vi "Color sensor - main.vi"() -> ()   [LabVIEW 2022 SP3]
uses:
  Power mode.ctl
panel:
  in  "RED MIN 2%":dbl=193.0
  in  "RED MAX 2%":dbl=1715.0
  in  "BLUE MIN 2%":dbl=221.0
  in  "GREEN MIN 2%":dbl=158.0
  in  "GREEN MAX 2%":dbl=1834.0
  in  "BLUE MAX 2%":dbl=2778.0
  in  "RED MIN 20%":dbl=1939.0
  in  "RED MAX 20%":dbl=17200.0
  in  "BLUE MIN 20%":dbl=2215.0
  in  "GREEN MIN 20%":dbl=1585.0
  in  "GREEN MAX 20%":dbl=18400.0
  in  "BLUE MAX 20%":dbl=27800.0
  in  "Power mode":T1=enum."100%"
  in  "GREEN Sensitivity":dbl(slide)=1.0 scale=0.0..2.0
  in  "BLUE Sensitivity":dbl(slide)=1.0 scale=0.0..2.0
  in  "RED Sensitivity":dbl(slide)=1.0 scale=0.0..2.0
  in  "RGB TARGET":u32(colorbox)=16448250
  out "TARGET B":dbl=250.0 caption="B" format="%#_3g"
  out "TARGET G":dbl=250.0 caption="G" format="%#_3g"
  out "TARGET R":dbl=250.0 caption="R" format="%#_3g"
  out "G":dbl format="%#_3g"
  out "R":dbl format="%#_3g"
  out "B":dbl format="%#_3g"
  in  "GREEN MAX 100%":dbl=92000.0
  in  "GREEN MIN 100%":dbl=7910.0
  in  "BLUE MAX 100%":dbl=139000.0
  in  "BLUE MIN 100%":dbl=11060.0
  in  "RED MAX 100%":dbl=85900.0
  in  "RED MIN 100%":dbl=9680.0
  out "RGB OUTPUT":u32(colorbox)=262914
  out "GREEN Frequency":dbl
  out "CLEAR Frequency":dbl
  out "BLUE Frequency":dbl
  in  "stop":bool
  out "RED Frequency":dbl
  out "Color Chart":T2(graph)={"Scalar"=10835.410120273053, "Scalar"=12236.906510034263, "Scalar"=31123.560535325243, "Scalar"=8833.141948591114}
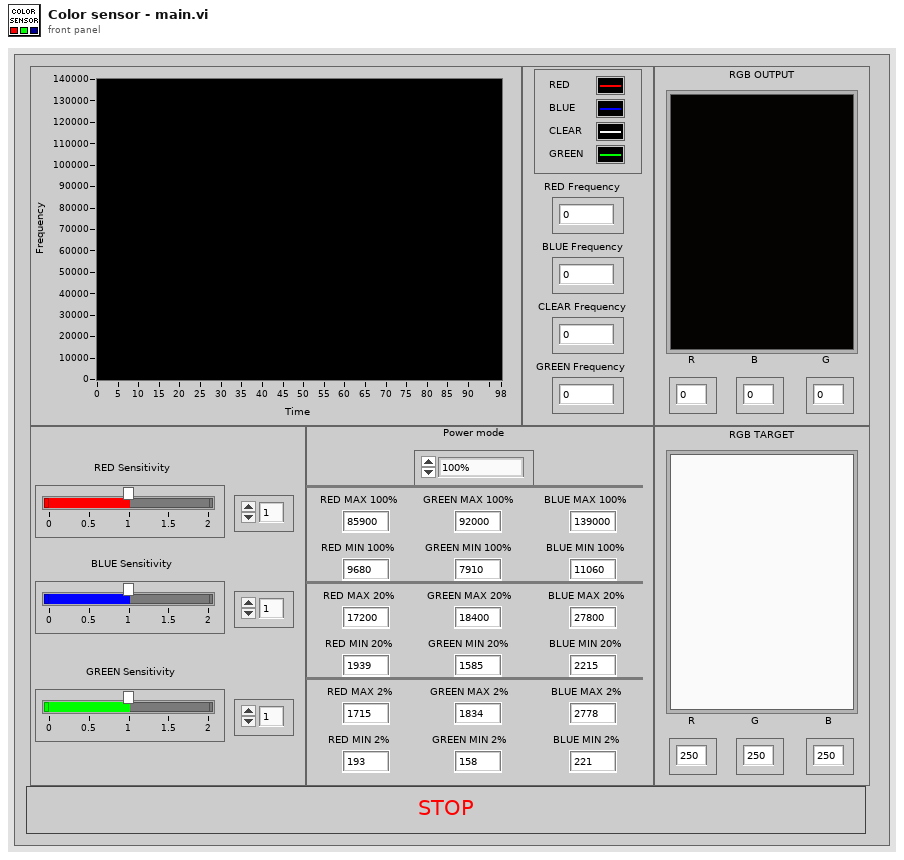
[diagram p1: front panel]
types:
  T1 = typedef "Power mode.ctl" = enum16{"Power down", "2%", "20%", "100%"}
  T2 = cluster{"Scalar":dbl, "Scalar":dbl, "Scalar":dbl, "Scalar":dbl}
  T3 = cluster{"Scalar":dbl, "Scalar":dbl, "Scalar":dbl, "Scalar":dbl}[]
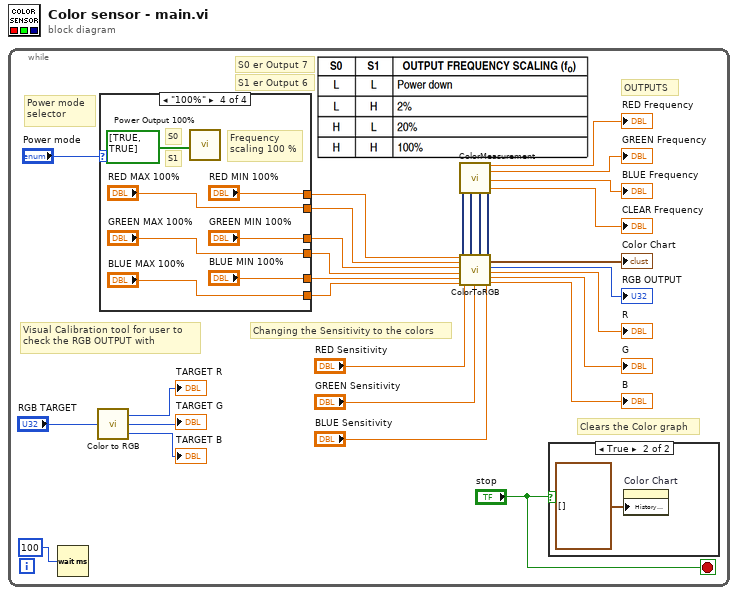
[diagram p0: block diagram]
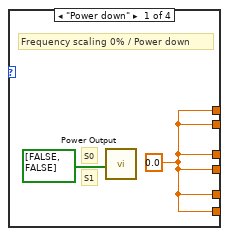
[diagram p3: hidden frame]
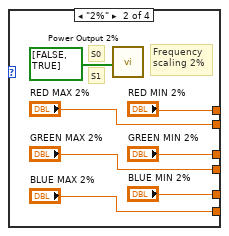
[diagram p4: hidden frame]
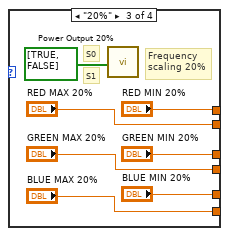
[diagram p5: hidden frame]
diagram:
  n1 = while {
    stop <- "stop" stop-if-true
    # "S1 er Output 6"
    # "S0 er Output 7"
    # "Power mode\nselector"
    # "OUTPUTS"
    # "Clears the Color graph"
    # "Changing the Sensitivity to the colors"
    # "Visual Calibration tool for user to \ncheck the RGB OUTPUT with"
    n2 = Wait (ms)(milliseconds to wait=u32 100) -> ()  [unwired: 1 out]
    n3 = call <vilib>:"Color to RGB.vi"("Color"="RGB TARGET") -> ("R"=→"TARGET R":u8, "G"=→"TARGET G":u8, "B"=→"TARGET B":u8)  [unwired: 1 out]
    n4 = case shown="\"100%\"" "Power mode" {
      tunnel: [w32 "GREEN MAX 2%" "GREEN MAX 20%" "GREEN MAX 100%"] -> w22
      tunnel: [w32 "GREEN MIN 2%" "GREEN MIN 20%" "GREEN MIN 100%"] -> w21
      tunnel: [w32 "BLUE MIN 2%" "BLUE MIN 20%" "BLUE MIN 100%"] -> w20
      tunnel: [w32 "RED MAX 2%" "RED MAX 20%" "RED MAX 100%"] -> w12
      tunnel: [w32 "RED MIN 2%" "RED MIN 20%" "RED MIN 100%"] -> w19
      tunnel: [w32 "BLUE MAX 2%" "BLUE MAX 20%" "BLUE MAX 100%"] -> w18
      frame "Power down" {
        w32 = 0.0 ("RED MIN 100%")
        # "S1"
        # "S0"
        # "Frequency scaling 0% / Power down"
        n5 = call "Power Output"("data"=bool[] [FALSE, FALSE]) -> ()  [unwired: 17 in, 2 out]
      }
      frame "2%" {
        # "S1"
        # "S0"
        # "Frequency \nscaling 2%"
        n6 = call "Power Output 2%"("data"=bool[] [FALSE, TRUE]) -> ()  [unwired: 17 in, 2 out]
      }
      frame "20%" {
        # "S1"
        # "S0"
        # "Frequency \nscaling 20%"
        n7 = call "Power Output 20%"("data"=bool[] [TRUE, FALSE]) -> ()  [unwired: 17 in, 2 out]
      }
      frame "100%" {
        # "S1"
        # "S0"
        # "Frequency\nscaling 100 %"
        n8 = call "Power Output 100%"("data"=bool[] [TRUE, TRUE]) -> ()  [unwired: 17 in, 2 out]
      }
    }
    n9 = call "ColorMeasurement.vi"() -> ("CLEAR INPUT"=w27:dynamicdata, "GREEN INPUT"=w17:dynamicdata, "CLEAR Frequency"=→"CLEAR Frequency":dbl, "GREEN Frequency"=→"GREEN Frequency":dbl, "BLUE INPUT"=w16:dynamicdata, "RED Frequency"=→"RED Frequency":dbl, "RED INPUT"=w28:dynamicdata, "BLUE Frequency"=→"BLUE Frequency":dbl)  [unwired: 4 in]
    n10 = call "ColorToRGB.vi"("RED INPUT"=w28, "RED MIN"=w19, "RED MAX"=w12, "GREEN MIN"=w21, "GREEN MAX"=w22, "BLUE INPUT"=w16, "BLUE MIN"=w20, "GREEN Sensitivity"="GREEN Sensitivity", "BLUE MAX"=w18, "CLEAR INPUT"=w27, "RED Sensitivity"="RED Sensitivity", "GREEN INPUT"=w17, "BLUE Sensitivity"="BLUE Sensitivity") -> ("G"=→"G":dbl, "SENSOR OUTPUT"=→"RGB OUTPUT":u32, "B"=→"B":dbl, "Color Chart"=→"Color Chart":T2, "R"=→"R":dbl)  [unwired: 2 in]
    n11 = case shown="True" "stop" {
      frame False {
      }
      frame True {
        n12 = property on="Color Chart" class="WFChart (strict)"("History Data"=T3 []) -> ()  [unwired: 2 in, 2 out]
      }
    }
  }
